vi "multimeterp1.vi"() -> ()   [LabVIEW 2013]
panel:
  in  "Continious \nMeasure":bool
  in  "Measure":bool
  out "Results, V":string[](array[string])
  in  "Range-":bool
  in  "Range+":bool
  out "error out":errorcluster
  in  "Mode":T1(radio)
  out "Range MAX":dbl format="%#_13g"
  out "Range No":dbl format="%#_13g"
  in  "VISA Address":refnum<visa-resource-name>
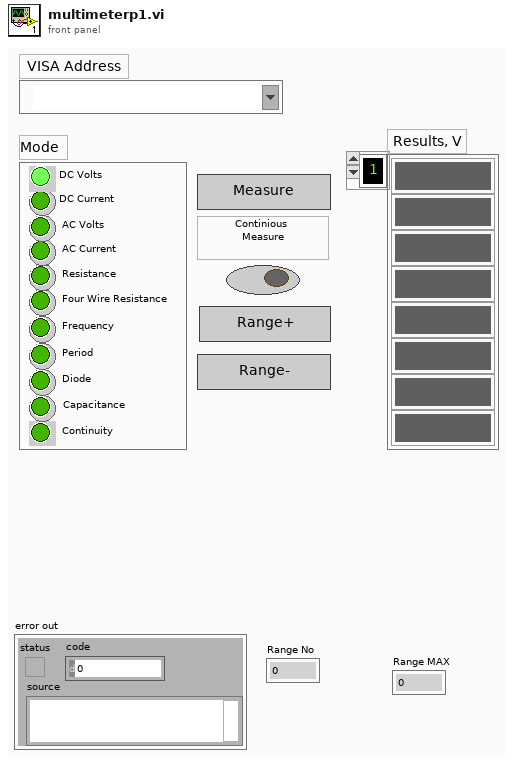
[diagram p1: front panel]
types:
  T1 = enum32{"DC Volts", "DC Current", "AC Volts", "AC Current", "Resistance", "Four Wire Resistance", "Frequency", "Period", "Diode", "Capacitance", "Continuity"}
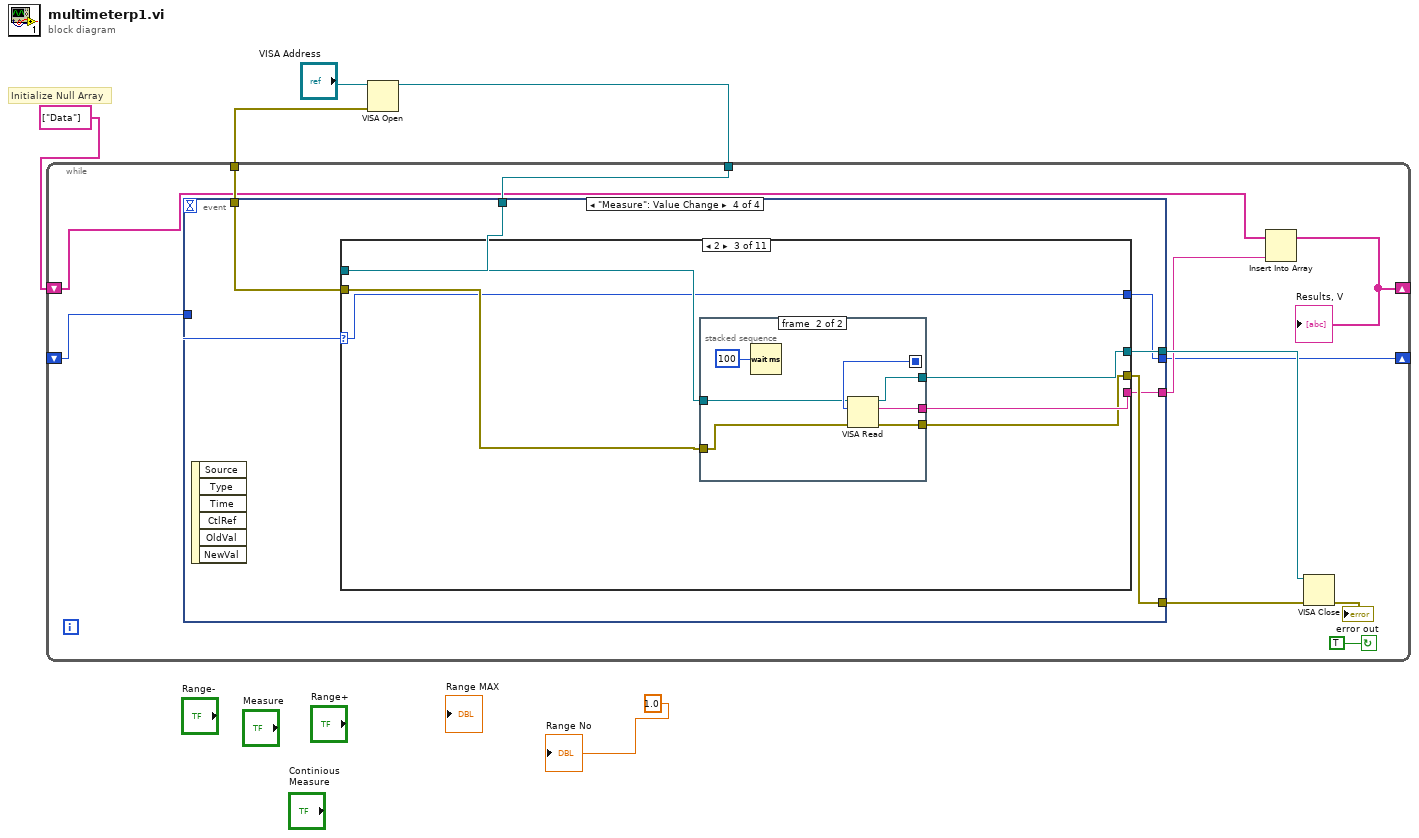
[diagram p0: block diagram]
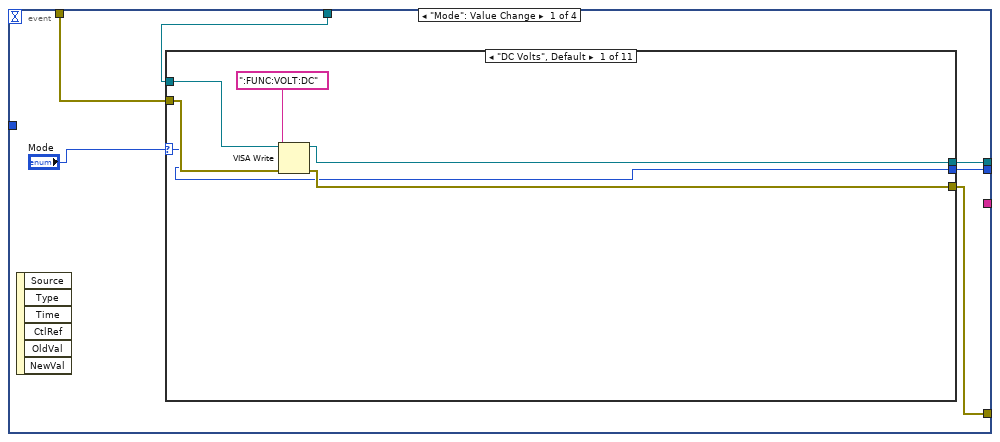
[diagram p2: hidden frame]
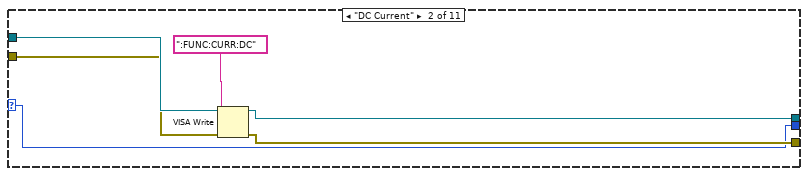
[diagram p3: hidden frame]
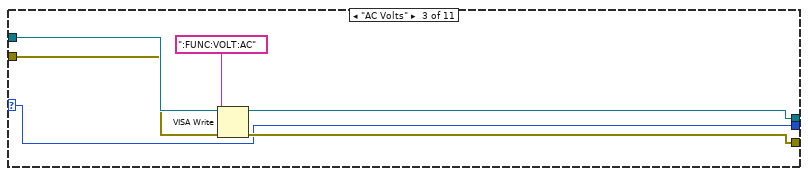
[diagram p4: hidden frame]
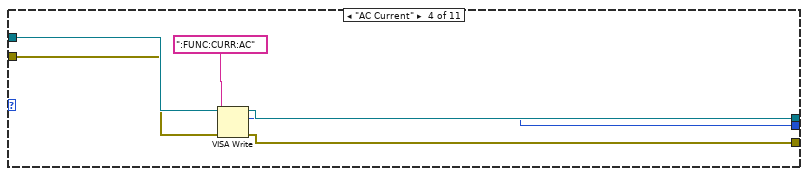
[diagram p5: hidden frame]
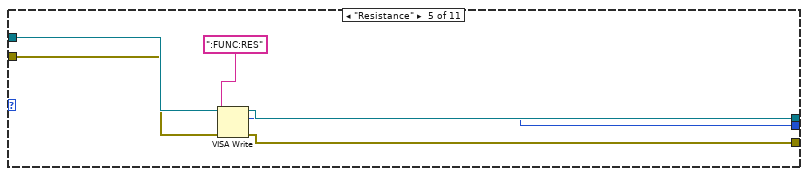
[diagram p6: hidden frame]
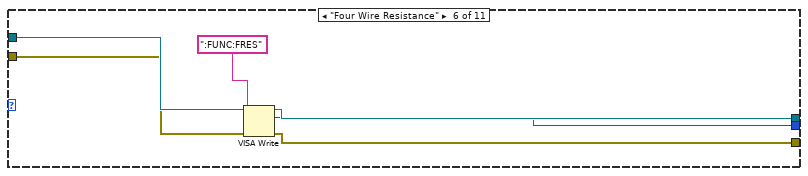
[diagram p7: hidden frame]
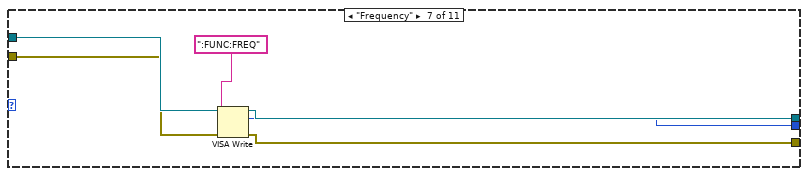
[diagram p8: hidden frame]
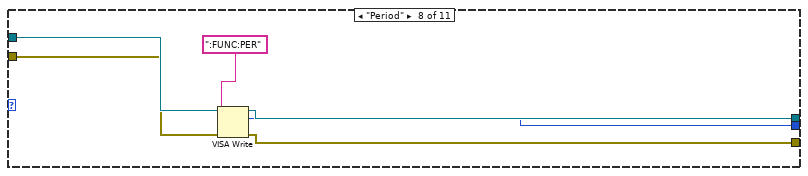
[diagram p9: hidden frame]
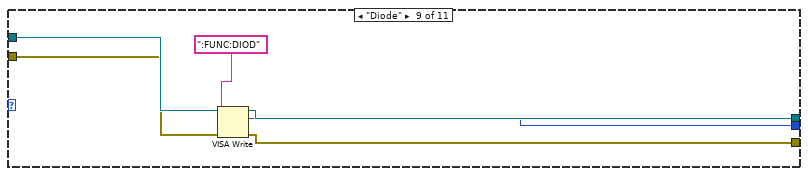
[diagram p10: hidden frame]
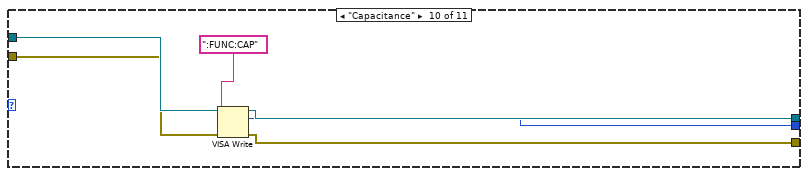
[diagram p11: hidden frame]
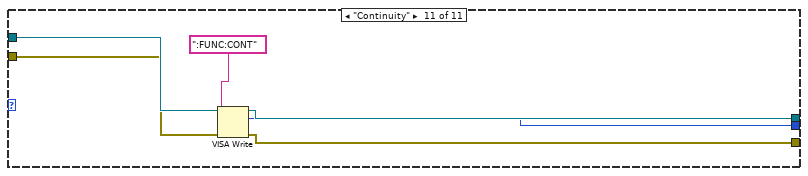
[diagram p12: hidden frame]
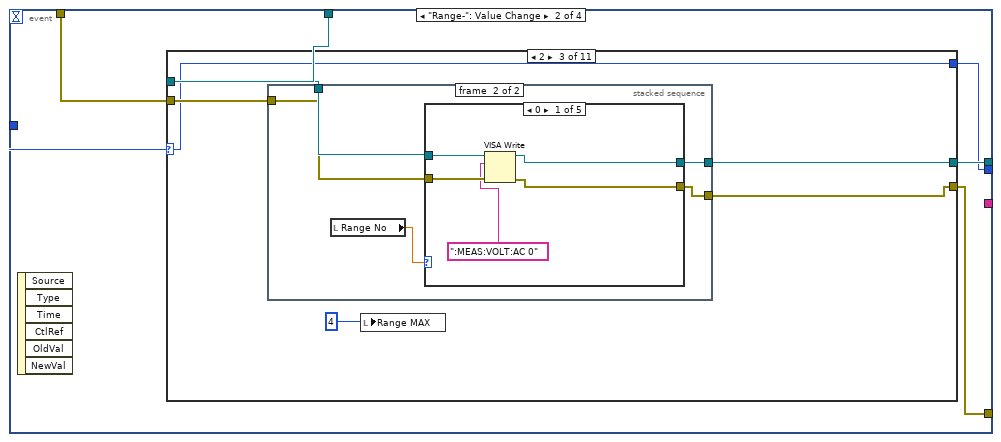
[diagram p13: hidden frame]
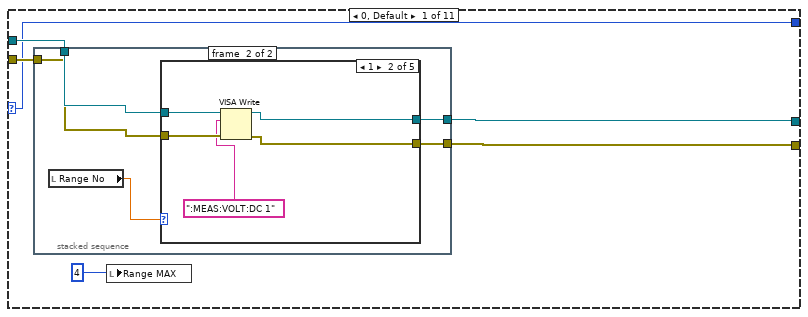
[diagram p14: hidden frame]
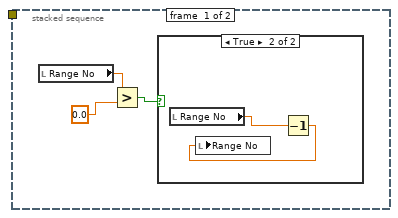
[diagram p15: hidden frame]
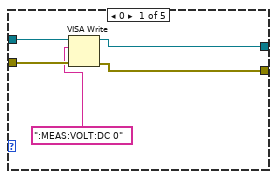
[diagram p17: hidden frame]
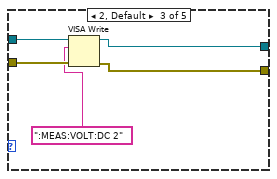
[diagram p18: hidden frame]
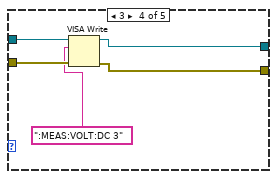
[diagram p19: hidden frame]
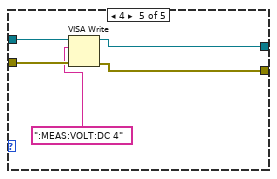
[diagram p20: hidden frame]
diagram:
  # "Initialize Null Array"
  n1 = VISA Open(VISA resource name="VISA Address") -> (VISA resource name=w2:refnum<visa-resource-name>, error out=w3:errorcluster)  [unwired: 4 in]
  n2 = while {
    tunnel: w3 -> [w14]
    tunnel: w2 -> [w13]
    shift-right: [w8] -> _
    shift-left: _ -> [w9]
    shift-right: [w7] -> _
    shift-left: string[] ["Data"] ("array") -> [w6]
    stop <- TRUE continue-if-true
    n3 = event shown="[3] \"Measure\": Value Change" {
      selector: _ -> [_ _ _ _]
      dyn-events: _ -> [_ _ _ _]
      timeout: _ -> [_ _ _ _]
      tunnel: w14 -> [w22 w94 w576 w1059]
      tunnel: w13 -> [w19 w91 w573 w1056]
      tunnel: [w21 w93 w575 w1058] -> w12
      tunnel: [w20 w92 w574 w1057] -> w11
      tunnel: [_ _ _ w1055] -> w10
      tunnel: w9 -> [_ w90 w572 w1054]
      tunnel: [w18 w89 w571 w1053] -> w8
      event "Mode": Value Change {
        n4 = event-data() -> ()  [unwired: 1 in, 6 out]
        n5 = case shown="\"DC Volts\", Default" "Mode" {
          selector: "Mode" -> [w23 w29 w35 _ _ _ _ _ _ _ _]
          tunnel: w19 -> [w26 w33 w39 w45 w51 w57 w63 w69 w75 w81 w87]
          tunnel: w22 -> [w27 w32 w38 w44 w50 w56 w62 w68 w74 w80 w86]
          tunnel: [w24 w30 w36 w42 w48 w54 w60 w66 w72 w78 w84] -> w21
          tunnel: [w25 w31 w37 w43 w49 w55 w61 w67 w73 w79 w85] -> w20
          tunnel: [w23 w29 w35 w41 w47 w53 w59 w65 w71 w77 w83] -> w18
          frame "DC Volts", Default {
            n6 = VISA Write(VISA resource name=w26, write buffer=":FUNC:VOLT:DC", error in (no error)=w27) -> (VISA resource name out=w25:refnum<visa-resource-name>, error out=w24:errorcluster)  [unwired: 1 out]
          }
          frame "DC Current" {
            n7 = VISA Write(VISA resource name=w33, write buffer=":FUNC:CURR:DC", error in (no error)=w32) -> (VISA resource name out=w31:refnum<visa-resource-name>, error out=w30:errorcluster)  [unwired: 1 out]
          }
          frame "AC Volts" {
            n8 = VISA Write(VISA resource name=w39, write buffer=":FUNC:VOLT:AC", error in (no error)=w38) -> (VISA resource name out=w37:refnum<visa-resource-name>, error out=w36:errorcluster)  [unwired: 1 out]
          }
          frame "AC Current" {
            n9 = VISA Write(VISA resource name=w45, write buffer=":FUNC:CURR:AC", error in (no error)=w44) -> (VISA resource name out=w43:refnum<visa-resource-name>, return count=w41:u32, error out=w42:errorcluster)
          }
          frame "Resistance" {
            n10 = VISA Write(VISA resource name=w51, write buffer=":FUNC:RES", error in (no error)=w50) -> (VISA resource name out=w49:refnum<visa-resource-name>, return count=w47:u32, error out=w48:errorcluster)
          }
          frame "Four Wire Resistance" {
            n11 = VISA Write(VISA resource name=w57, write buffer=":FUNC:FRES", error in (no error)=w56) -> (VISA resource name out=w55:refnum<visa-resource-name>, return count=w53:u32, error out=w54:errorcluster)
          }
          frame "Frequency" {
            n12 = VISA Write(VISA resource name=w63, write buffer=":FUNC:FREQ", error in (no error)=w62) -> (VISA resource name out=w61:refnum<visa-resource-name>, return count=w59:u32, error out=w60:errorcluster)
          }
          frame "Period" {
            n13 = VISA Write(VISA resource name=w69, write buffer=":FUNC:PER", error in (no error)=w68) -> (VISA resource name out=w67:refnum<visa-resource-name>, return count=w65:u32, error out=w66:errorcluster)
          }
          frame "Diode" {
            n14 = VISA Write(VISA resource name=w75, write buffer=":FUNC:DIOD", error in (no error)=w74) -> (VISA resource name out=w73:refnum<visa-resource-name>, return count=w71:u32, error out=w72:errorcluster)
          }
          frame "Capacitance" {
            n15 = VISA Write(VISA resource name=w81, write buffer=":FUNC:CAP", error in (no error)=w80) -> (VISA resource name out=w79:refnum<visa-resource-name>, return count=w77:u32, error out=w78:errorcluster)
          }
          frame "Continuity" {
            n16 = VISA Write(VISA resource name=w87, write buffer=":FUNC:CONT", error in (no error)=w86) -> (VISA resource name out=w85:refnum<visa-resource-name>, return count=w83:u32, error out=w84:errorcluster)
          }
        }
      }
      event "Range-": Value Change {
        n17 = event-data() -> ()  [unwired: 1 in, 6 out]
        n18 = case shown="2" w90 {
          selector: w90 -> [w95 w136 w182 w223 w259 w310 w361 w402 w443 w484 w530]
          tunnel: w91 -> [w99 w138 w186 w227 w263 w314 w364 w405 w446 w485 w532]
          tunnel: w94 -> [w98 w137 w185 w226 w262 w313 w365 w406 w447 w486 w531]
          tunnel: [w96 w139 w183 w224 w261 w311 w362 w403 w444 w487 w533] -> w93
          tunnel: [w97 w140 w184 w225 w260 w312 w363 w404 w445 w488 w534] -> w92
          tunnel: [w95 w136 w182 w223 w259 w310 w361 w402 w443 w484 w530] -> w89
          frame 0, Default {
            n19 = stacked-sequence {
              tunnel: w99 -> [_ w109]
              tunnel: w98 -> [_ w108]
              tunnel: [_ w107] -> w97
              tunnel: [_ w106] -> w96
              frame #0 {
                n20 = local read "Range No"() -> (w102:dbl)
                n21 = Greater?(x=w102, y=0.0) -> (0:w101:bool)
                n22 = case shown="True" w101 {
                  frame False {
                  }
                  frame True {
                    n23 = local read "Range No"() -> (w104:dbl)
                    n24 = Decrement(x=w104) -> (x-1=w105:dbl)
                    n25 = local write "Range No"(w105) -> ()
                  }
                }
              }
              frame #1 {
                n26 = local read "Range No"() -> (w110:dbl)
                n27 = case shown="1" w110 {
                  tunnel: w109 -> [w115 w120 w125 w130 w135]
                  tunnel: w108 -> [w114 w119 w124 w129 w134]
                  tunnel: [w112 w117 w122 w127 w132] -> w107
                  tunnel: [w111 w116 w121 w126 w131] -> w106
                  frame 0 {
                    n28 = VISA Write(VISA resource name=w115, write buffer=":MEAS:VOLT:DC 0", error in (no error)=w114) -> (VISA resource name out=w112:refnum<visa-resource-name>, error out=w111:errorcluster)  [unwired: 1 out]
                  }
                  frame 1 {
                    n29 = VISA Write(VISA resource name=w120, write buffer=":MEAS:VOLT:DC 1", error in (no error)=w119) -> (VISA resource name out=w117:refnum<visa-resource-name>, error out=w116:errorcluster)  [unwired: 1 out]
                  }
                  frame 2, Default {
                    n30 = VISA Write(VISA resource name=w125, write buffer=":MEAS:VOLT:DC 2", error in (no error)=w124) -> (VISA resource name out=w122:refnum<visa-resource-name>, error out=w121:errorcluster)  [unwired: 1 out]
                  }
                  frame 3 {
                    n31 = VISA Write(VISA resource name=w130, write buffer=":MEAS:VOLT:DC 3", error in (no error)=w129) -> (VISA resource name out=w127:refnum<visa-resource-name>, error out=w126:errorcluster)  [unwired: 1 out]
                  }
                  frame 4 {
                    n32 = VISA Write(VISA resource name=w135, write buffer=":MEAS:VOLT:DC 4", error in (no error)=w134) -> (VISA resource name out=w132:refnum<visa-resource-name>, error out=w131:errorcluster)  [unwired: 1 out]
                  }
                }
              }
            }
            n33 = local write "Range MAX"(4) -> ()
          }
          frame 1 {
            n34 = stacked-sequence {
              tunnel: [_ w150] -> w140
              tunnel: [_ w149] -> w139
              tunnel: w138 -> [_ w148]
              tunnel: w137 -> [_ w147]
              frame #0 {
                n35 = local read "Range No"() -> (w143:dbl)
                n36 = Greater?(x=w143, y=0.0) -> (0:w142:bool)
                n37 = case shown="True" w142 {
                  frame False {
                  }
                  frame True {
                    n38 = local read "Range No"() -> (w145:dbl)
                    n39 = Decrement(x=w145) -> (x-1=w146:dbl)
                    n40 = local write "Range No"(w146) -> ()
                  }
                }
              }
              frame #1 {
                n41 = local read "Range No"() -> (w151:dbl)
                n42 = case shown="1" w151 {
                  tunnel: w148 -> [w156 w161 w166 w171 w176 w181]
                  tunnel: w147 -> [w155 w160 w165 w170 w175 w180]
                  tunnel: [w153 w158 w163 w168 w173 w178] -> w150
                  tunnel: [w152 w157 w162 w167 w172 w177] -> w149
                  frame 0 {
                    n43 = VISA Write(VISA resource name=w156, write buffer=":MEAS:CURR:DC 0", error in (no error)=w155) -> (VISA resource name out=w153:refnum<visa-resource-name>, error out=w152:errorcluster)  [unwired: 1 out]
                  }
                  frame 1 {
                    n44 = VISA Write(VISA resource name=w161, write buffer=":MEAS:CURR:DC 1", error in (no error)=w160) -> (VISA resource name out=w158:refnum<visa-resource-name>, error out=w157:errorcluster)  [unwired: 1 out]
                  }
                  frame 2, Default {
                    n45 = VISA Write(VISA resource name=w166, write buffer=":MEAS:CURR:DC 2", error in (no error)=w165) -> (VISA resource name out=w163:refnum<visa-resource-name>, error out=w162:errorcluster)  [unwired: 1 out]
                  }
                  frame 3 {
                    n46 = VISA Write(VISA resource name=w171, write buffer=":MEAS:CURR:DC 3", error in (no error)=w170) -> (VISA resource name out=w168:refnum<visa-resource-name>, error out=w167:errorcluster)  [unwired: 1 out]
                  }
                  frame 4 {
                    n47 = VISA Write(VISA resource name=w176, write buffer=":MEAS:CURR:DC 4", error in (no error)=w175) -> (VISA resource name out=w173:refnum<visa-resource-name>, error out=w172:errorcluster)  [unwired: 1 out]
                  }
                  frame 5 {
                    n48 = VISA Write(VISA resource name=w181, write buffer=":MEAS:CURR:DC 5", error in (no error)=w180) -> (VISA resource name out=w178:refnum<visa-resource-name>, error out=w177:errorcluster)  [unwired: 1 out]
                  }
                }
              }
            }
            n49 = local write "Range MAX"(5) -> ()
          }
          frame 2 {
            n50 = stacked-sequence {
              tunnel: w186 -> [_ w196]
              tunnel: w185 -> [_ w195]
              tunnel: [_ w194] -> w184
              tunnel: [_ w193] -> w183
              frame #0 {
                n51 = local read "Range No"() -> (w189:dbl)
                n52 = Greater?(x=w189, y=0.0) -> (0:w188:bool)
                n53 = case shown="True" w188 {
                  frame False {
                  }
                  frame True {
                    n54 = local read "Range No"() -> (w191:dbl)
                    n55 = Decrement(x=w191) -> (x-1=w192:dbl)
                    n56 = local write "Range No"(w192) -> ()
                  }
                }
              }
              frame #1 {
                n57 = local read "Range No"() -> (w197:dbl)
                n58 = case shown="0" w197 {
                  tunnel: w196 -> [w202 w207 w212 w217 w222]
                  tunnel: w195 -> [w201 w206 w211 w216 w221]
                  tunnel: [w199 w204 w209 w214 w219] -> w194
                  tunnel: [w198 w203 w208 w213 w218] -> w193
                  frame 0 {
                    n59 = VISA Write(VISA resource name=w202, write buffer=":MEAS:VOLT:AC 0", error in (no error)=w201) -> (VISA resource name out=w199:refnum<visa-resource-name>, error out=w198:errorcluster)  [unwired: 1 out]
                  }
                  frame 1 {
                    n60 = VISA Write(VISA resource name=w207, write buffer=":MEAS:VOLT:AC 1", error in (no error)=w206) -> (VISA resource name out=w204:refnum<visa-resource-name>, error out=w203:errorcluster)  [unwired: 1 out]
                  }
                  frame 2, Default {
                    n61 = VISA Write(VISA resource name=w212, write buffer=":MEAS:VOLT:AC 2", error in (no error)=w211) -> (VISA resource name out=w209:refnum<visa-resource-name>, error out=w208:errorcluster)  [unwired: 1 out]
                  }
                  frame 3 {
                    n62 = VISA Write(VISA resource name=w217, write buffer=":MEAS:VOLT:AC 3", error in (no error)=w216) -> (VISA resource name out=w214:refnum<visa-resource-name>, error out=w213:errorcluster)  [unwired: 1 out]
                  }
                  frame 4 {
                    n63 = VISA Write(VISA resource name=w222, write buffer=":MEAS:VOLT:AC 4", error in (no error)=w221) -> (VISA resource name out=w219:refnum<visa-resource-name>, error out=w218:errorcluster)  [unwired: 1 out]
                  }
                }
              }
            }
            n64 = local write "Range MAX"(4) -> ()
          }
          frame 3 {
            n65 = stacked-sequence {
              tunnel: w227 -> [_ w237]
              tunnel: w226 -> [_ w236]
              tunnel: [_ w235] -> w225
              tunnel: [_ w234] -> w224
              frame #0 {
                n66 = local read "Range No"() -> (w230:dbl)
                n67 = Greater?(x=w230, y=0.0) -> (0:w229:bool)
                n68 = case shown="True" w229 {
                  frame False {
                  }
                  frame True {
                    n69 = local read "Range No"() -> (w232:dbl)
                    n70 = Decrement(x=w232) -> (x-1=w233:dbl)
                    n71 = local write "Range No"(w233) -> ()
                  }
                }
              }
              frame #1 {
                n72 = local read "Range No"() -> (w238:dbl)
                n73 = case shown="0" w238 {
                  tunnel: w237 -> [w243 w248 w253 w258]
                  tunnel: w236 -> [w242 w247 w252 w257]
                  tunnel: [w240 w245 w250 w255] -> w235
                  tunnel: [w239 w244 w249 w254] -> w234
                  frame 0 {
                    n74 = VISA Write(VISA resource name=w243, write buffer=":MEAS:CURR:AC 0", error in (no error)=w242) -> (VISA resource name out=w240:refnum<visa-resource-name>, error out=w239:errorcluster)  [unwired: 1 out]
                  }
                  frame 1 {
                    n75 = VISA Write(VISA resource name=w248, write buffer=":MEAS:CURR:AC 1", error in (no error)=w247) -> (VISA resource name out=w245:refnum<visa-resource-name>, error out=w244:errorcluster)  [unwired: 1 out]
                  }
                  frame 2, Default {
                    n76 = VISA Write(VISA resource name=w253, write buffer=":MEAS:CURR:AC 2", error in (no error)=w252) -> (VISA resource name out=w250:refnum<visa-resource-name>, error out=w249:errorcluster)  [unwired: 1 out]
                  }
                  frame 3 {
                    n77 = VISA Write(VISA resource name=w258, write buffer=":MEAS:CURR:AC 3", error in (no error)=w257) -> (VISA resource name out=w255:refnum<visa-resource-name>, error out=w254:errorcluster)  [unwired: 1 out]
                  }
                }
              }
            }
            n78 = local write "Range MAX"(3) -> ()
          }
          frame 4 {
            n79 = stacked-sequence {
              tunnel: w263 -> [_ w273]
              tunnel: w262 -> [_ w272]
              tunnel: [_ w271] -> w261
              tunnel: [_ w270] -> w260
              frame #0 {
                n80 = local read "Range No"() -> (w266:dbl)
                n81 = Greater?(x=w266, y=0.0) -> (0:w265:bool)
                n82 = case shown="True" w265 {
                  frame False {
                  }
                  frame True {
                    n83 = local read "Range No"() -> (w268:dbl)
                    n84 = Decrement(x=w268) -> (x-1=w269:dbl)
                    n85 = local write "Range No"(w269) -> ()
                  }
                }
              }
              frame #1 {
                n86 = local read "Range No"() -> (w274:dbl)
                n87 = case shown="1" w274 {
                  tunnel: w273 -> [w279 w284 w289 w294 w299 w304 w309]
                  tunnel: w272 -> [w278 w283 w288 w293 w298 w303 w308]
                  tunnel: [w276 w281 w286 w291 w296 w301 w306] -> w270
                  tunnel: [w275 w280 w285 w290 w295 w300 w305] -> w271
                  frame 0 {
                    n88 = VISA Write(VISA resource name=w279, write buffer=":MEAS:RES 0", error in (no error)=w278) -> (VISA resource name out=w276:refnum<visa-resource-name>, error out=w275:errorcluster)  [unwired: 1 out]
                  }
                  frame 1 {
                    n89 = VISA Write(VISA resource name=w284, write buffer=":MEAS:RES 1", error in (no error)=w283) -> (VISA resource name out=w281:refnum<visa-resource-name>, error out=w280:errorcluster)  [unwired: 1 out]
                  }
                  frame 2, Default {
                    n90 = VISA Write(VISA resource name=w289, write buffer=":MEAS:RES 2", error in (no error)=w288) -> (VISA resource name out=w286:refnum<visa-resource-name>, error out=w285:errorcluster)  [unwired: 1 out]
                  }
                  frame 3 {
                    n91 = VISA Write(VISA resource name=w294, write buffer=":MEAS:RES 3", error in (no error)=w293) -> (VISA resource name out=w291:refnum<visa-resource-name>, error out=w290:errorcluster)  [unwired: 1 out]
                  }
                  frame 4 {
                    n92 = VISA Write(VISA resource name=w299, write buffer=":MEAS:RES 4", error in (no error)=w298) -> (VISA resource name out=w296:refnum<visa-resource-name>, error out=w295:errorcluster)  [unwired: 1 out]
                  }
                  frame 5 {
                    n93 = VISA Write(VISA resource name=w304, write buffer=":MEAS:RES 5", error in (no error)=w303) -> (VISA resource name out=w301:refnum<visa-resource-name>, error out=w300:errorcluster)  [unwired: 1 out]
                  }
                  frame 6 {
                    n94 = VISA Write(VISA resource name=w309, write buffer=":MEAS:RES 6", error in (no error)=w308) -> (VISA resource name out=w306:refnum<visa-resource-name>, error out=w305:errorcluster)  [unwired: 1 out]
                  }
                }
              }
            }
            n95 = local write "Range MAX"(6) -> ()
          }
          frame 5 {
            n96 = stacked-sequence {
              tunnel: w314 -> [_ w324]
              tunnel: w313 -> [_ w323]
              tunnel: [_ w322] -> w312
              tunnel: [_ w321] -> w311
              frame #0 {
                n97 = local read "Range No"() -> (w317:dbl)
                n98 = Greater?(x=w317, y=0.0) -> (0:w316:bool)
                n99 = case shown="True" w316 {
                  frame False {
                  }
                  frame True {
                    n100 = local read "Range No"() -> (w319:dbl)
                    n101 = Decrement(x=w319) -> (x-1=w320:dbl)
                    n102 = local write "Range No"(w320) -> ()
                  }
                }
              }
              frame #1 {
                n103 = local read "Range No"() -> (w325:dbl)
                n104 = case shown="6" w325 {
                  tunnel: w324 -> [w330 w335 w340 w345 w350 w355 w360]
                  tunnel: w323 -> [w329 w334 w339 w344 w349 w354 w359]
                  tunnel: [w327 w332 w337 w342 w347 w352 w357] -> w322
                  tunnel: [w326 w331 w336 w341 w346 w351 w356] -> w321
                  frame 0 {
                    n105 = VISA Write(VISA resource name=w330, write buffer=":MEAS:FRES 0", error in (no error)=w329) -> (VISA resource name out=w327:refnum<visa-resource-name>, error out=w326:errorcluster)  [unwired: 1 out]
                  }
                  frame 1 {
                    n106 = VISA Write(VISA resource name=w335, write buffer=":MEAS:FRES 1", error in (no error)=w334) -> (VISA resource name out=w332:refnum<visa-resource-name>, error out=w331:errorcluster)  [unwired: 1 out]
                  }
                  frame 2, Default {
                    n107 = VISA Write(VISA resource name=w340, write buffer=":MEAS:FRES 2", error in (no error)=w339) -> (VISA resource name out=w337:refnum<visa-resource-name>, error out=w336:errorcluster)  [unwired: 1 out]
                  }
                  frame 3 {
                    n108 = VISA Write(VISA resource name=w345, write buffer=":MEAS:FRES 3", error in (no error)=w344) -> (VISA resource name out=w342:refnum<visa-resource-name>, error out=w341:errorcluster)  [unwired: 1 out]
                  }
                  frame 4 {
                    n109 = VISA Write(VISA resource name=w350, write buffer=":MEAS:FRES 4", error in (no error)=w349) -> (VISA resource name out=w347:refnum<visa-resource-name>, error out=w346:errorcluster)  [unwired: 1 out]
                  }
                  frame 5 {
                    n110 = VISA Write(VISA resource name=w355, write buffer=":MEAS:FRES 5", error in (no error)=w354) -> (VISA resource name out=w352:refnum<visa-resource-name>, error out=w351:errorcluster)  [unwired: 1 out]
                  }
                  frame 6 {
                    n111 = VISA Write(VISA resource name=w360, write buffer=":MEAS:FRES 6", error in (no error)=w359) -> (VISA resource name out=w357:refnum<visa-resource-name>, error out=w356:errorcluster)  [unwired: 1 out]
                  }
                }
              }
            }
            n112 = local write "Range MAX"(6) -> ()
          }
          frame 6 {
            n113 = stacked-sequence {
              tunnel: w365 -> [_ w375]
              tunnel: w364 -> [_ w374]
              tunnel: [_ w373] -> w363
              tunnel: [_ w372] -> w362
              frame #0 {
                n114 = local read "Range No"() -> (w368:dbl)
                n115 = Greater?(x=w368, y=0.0) -> (0:w367:bool)
                n116 = case shown="True" w367 {
                  frame False {
                  }
                  frame True {
                    n117 = local read "Range No"() -> (w370:dbl)
                    n118 = Decrement(x=w370) -> (x-1=w371:dbl)
                    n119 = local write "Range No"(w371) -> ()
                  }
                }
              }
              frame #1 {
                n120 = local read "Range No"() -> (w376:dbl)
                n121 = case shown="1" w376 {
                  tunnel: w374 -> [w381 w386 w391 w396 w401]
                  tunnel: w375 -> [w380 w385 w390 w395 w400]
                  tunnel: [w378 w383 w388 w393 w398] -> w373
                  tunnel: [w377 w382 w387 w392 w397] -> w372
                  frame 0 {
                    n122 = VISA Write(VISA resource name=w381, write buffer=":MEAS:FREQ 0", error in (no error)=w380) -> (VISA resource name out=w378:refnum<visa-resource-name>, error out=w377:errorcluster)  [unwired: 1 out]
                  }
                  frame 1 {
                    n123 = VISA Write(VISA resource name=w386, write buffer=":MEAS:FREQ 1", error in (no error)=w385) -> (VISA resource name out=w383:refnum<visa-resource-name>, error out=w382:errorcluster)  [unwired: 1 out]
                  }
                  frame 2, Default {
                    n124 = VISA Write(VISA resource name=w391, write buffer=":MEAS:FREQ 2", error in (no error)=w390) -> (VISA resource name out=w388:refnum<visa-resource-name>, error out=w387:errorcluster)  [unwired: 1 out]
                  }
                  frame 3 {
                    n125 = VISA Write(VISA resource name=w396, write buffer=":MEAS:FREQ 3", error in (no error)=w395) -> (VISA resource name out=w393:refnum<visa-resource-name>, error out=w392:errorcluster)  [unwired: 1 out]
                  }
                  frame 4 {
                    n126 = VISA Write(VISA resource name=w401, write buffer=":MEAS:FREQ 4", error in (no error)=w400) -> (VISA resource name out=w398:refnum<visa-resource-name>, error out=w397:errorcluster)  [unwired: 1 out]
                  }
                }
              }
            }
            n127 = local write "Range MAX"(4) -> ()
          }
          frame 7 {
            n128 = stacked-sequence {
              tunnel: w406 -> [_ w416]
              tunnel: w405 -> [_ w415]
              tunnel: [_ w414] -> w404
              tunnel: [_ w413] -> w403
              frame #0 {
                n129 = local read "Range No"() -> (w409:dbl)
                n130 = Greater?(x=w409, y=0.0) -> (0:w408:bool)
                n131 = case shown="True" w408 {
                  frame False {
                  }
                  frame True {
                    n132 = local read "Range No"() -> (w411:dbl)
                    n133 = Decrement(x=w411) -> (x-1=w412:dbl)
                    n134 = local write "Range No"(w412) -> ()
                  }
                }
              }
              frame #1 {
                n135 = local read "Range No"() -> (w417:dbl)
                n136 = case shown="0" w417 {
                  tunnel: w415 -> [w422 w427 w432 w437 w442]
                  tunnel: w416 -> [w421 w426 w431 w436 w441]
                  tunnel: [w419 w424 w429 w434 w439] -> w414
                  tunnel: [w418 w423 w428 w433 w438] -> w413
                  frame 0 {
                    n137 = VISA Write(VISA resource name=w422, write buffer=":MEAS:PER 0", error in (no error)=w421) -> (VISA resource name out=w419:refnum<visa-resource-name>, error out=w418:errorcluster)  [unwired: 1 out]
                  }
                  frame 1 {
                    n138 = VISA Write(VISA resource name=w427, write buffer=":MEAS:PER 1", error in (no error)=w426) -> (VISA resource name out=w424:refnum<visa-resource-name>, error out=w423:errorcluster)  [unwired: 1 out]
                  }
                  frame 2, Default {
                    n139 = VISA Write(VISA resource name=w432, write buffer=":MEAS:PER 2", error in (no error)=w431) -> (VISA resource name out=w429:refnum<visa-resource-name>, error out=w428:errorcluster)  [unwired: 1 out]
                  }
                  frame 3 {
                    n140 = VISA Write(VISA resource name=w437, write buffer=":MEAS:PER 3", error in (no error)=w436) -> (VISA resource name out=w434:refnum<visa-resource-name>, error out=w433:errorcluster)  [unwired: 1 out]
                  }
                  frame 4 {
                    n141 = VISA Write(VISA resource name=w442, write buffer=":MEAS:PER 4", error in (no error)=w441) -> (VISA resource name out=w439:refnum<visa-resource-name>, error out=w438:errorcluster)  [unwired: 1 out]
                  }
                }
              }
            }
            n142 = local write "Range MAX"(4) -> ()
          }
          frame 8 {
            n143 = stacked-sequence {
              tunnel: w447 -> [_ w457]
              tunnel: w446 -> [_ w456]
              tunnel: [_ w455] -> w445
              tunnel: [_ w454] -> w444
              frame #0 {
                n144 = local read "Range No"() -> (w450:dbl)
                n145 = Greater?(x=w450, y=0.0) -> (0:w449:bool)
                n146 = case shown="True" w449 {
                  frame False {
                  }
                  frame True {
                    n147 = local read "Range No"() -> (w452:dbl)
                    n148 = Decrement(x=w452) -> (x-1=w453:dbl)
                    n149 = local write "Range No"(w453) -> ()
                  }
                }
              }
              frame #1 {
                n150 = local read "Range No"() -> (w458:dbl)
                n151 = case shown="0" w458 {
                  tunnel: w456 -> [w463 w468 w473 w478 w483]
                  tunnel: w457 -> [w462 w467 w472 w477 w482]
                  tunnel: [w460 w465 w470 w475 w480] -> w455
                  tunnel: [w459 w464 w469 w474 w479] -> w454
                  frame 0 {
                    n152 = VISA Write(VISA resource name=w463, write buffer=":MEAS:VOLT:DC 0", error in (no error)=w462) -> (VISA resource name out=w460:refnum<visa-resource-name>, error out=w459:errorcluster)  [unwired: 1 out]
                  }
                  frame 1 {
                    n153 = VISA Write(VISA resource name=w468, write buffer=":MEAS:VOLT:DC 1", error in (no error)=w467) -> (VISA resource name out=w465:refnum<visa-resource-name>, error out=w464:errorcluster)  [unwired: 1 out]
                  }
                  frame 2, Default {
                    n154 = VISA Write(VISA resource name=w473, write buffer=":MEAS:VOLT:DC 2", error in (no error)=w472) -> (VISA resource name out=w470:refnum<visa-resource-name>, error out=w469:errorcluster)  [unwired: 1 out]
                  }
                  frame 3 {
                    n155 = VISA Write(VISA resource name=w478, write buffer=":MEAS:VOLT:DC 3", error in (no error)=w477) -> (VISA resource name out=w475:refnum<visa-resource-name>, error out=w474:errorcluster)  [unwired: 1 out]
                  }
                  frame 4 {
                    n156 = VISA Write(VISA resource name=w483, write buffer=":MEAS:VOLT:DC 4", error in (no error)=w482) -> (VISA resource name out=w480:refnum<visa-resource-name>, error out=w479:errorcluster)  [unwired: 1 out]
                  }
                }
              }
            }
            n157 = local write "Range MAX"(4) -> ()
          }
          frame 9 {
            n158 = stacked-sequence {
              tunnel: [_ w498] -> w488
              tunnel: [_ w497] -> w487
              tunnel: w486 -> [_ w496]
              tunnel: w485 -> [_ w495]
              frame #0 {
                n159 = local read "Range No"() -> (w491:dbl)
                n160 = Greater?(x=w491, y=0.0) -> (0:w490:bool)
                n161 = case shown="True" w490 {
                  frame False {
                  }
                  frame True {
                    n162 = local read "Range No"() -> (w493:dbl)
                    n163 = Decrement(x=w493) -> (x-1=w494:dbl)
                    n164 = local write "Range No"(w494) -> ()
                  }
                }
              }
              frame #1 {
                n165 = local read "Range No"() -> (w499:dbl)
                n166 = case shown="5" w499 {
                  tunnel: w495 -> [w504 w509 w514 w519 w524 w529]
                  tunnel: w496 -> [w503 w508 w513 w518 w523 w528]
                  tunnel: [w501 w506 w511 w516 w521 w526] -> w498
                  tunnel: [w500 w505 w510 w515 w520 w525] -> w497
                  frame 0 {
                    n167 = VISA Write(VISA resource name=w504, write buffer=":MEAS:CAP 0", error in (no error)=w503) -> (VISA resource name out=w501:refnum<visa-resource-name>, error out=w500:errorcluster)  [unwired: 1 out]
                  }
                  frame 1 {
                    n168 = VISA Write(VISA resource name=w509, write buffer=":MEAS:CAP 1", error in (no error)=w508) -> (VISA resource name out=w506:refnum<visa-resource-name>, error out=w505:errorcluster)  [unwired: 1 out]
                  }
                  frame 2, Default {
                    n169 = VISA Write(VISA resource name=w514, write buffer=":MEAS:CAP 2", error in (no error)=w513) -> (VISA resource name out=w511:refnum<visa-resource-name>, error out=w510:errorcluster)  [unwired: 1 out]
                  }
                  frame 3 {
                    n170 = VISA Write(VISA resource name=w519, write buffer=":MEAS:CAP 3", error in (no error)=w518) -> (VISA resource name out=w516:refnum<visa-resource-name>, error out=w515:errorcluster)  [unwired: 1 out]
                  }
                  frame 4 {
                    n171 = VISA Write(VISA resource name=w524, write buffer=":MEAS:CAP 4", error in (no error)=w523) -> (VISA resource name out=w521:refnum<visa-resource-name>, error out=w520:errorcluster)  [unwired: 1 out]
                  }
                  frame 5 {
                    n172 = VISA Write(VISA resource name=w529, write buffer=":MEAS:CAP 5", error in (no error)=w528) -> (VISA resource name out=w526:refnum<visa-resource-name>, error out=w525:errorcluster)  [unwired: 1 out]
                  }
                }
              }
            }
            n173 = local write "Range MAX"(5) -> ()
          }
          frame 10 {
            n174 = stacked-sequence {
              tunnel: [_ w544] -> w534
              tunnel: [_ w543] -> w533
              tunnel: w532 -> [_ w542]
              tunnel: w531 -> [_ w541]
              frame #0 {
                n175 = local read "Range No"() -> (w537:dbl)
                n176 = Greater?(x=w537, y=0.0) -> (0:w536:bool)
                n177 = case shown="True" w536 {
                  frame False {
                  }
                  frame True {
                    n178 = local read "Range No"() -> (w539:dbl)
                    n179 = Decrement(x=w539) -> (x-1=w540:dbl)
                    n180 = local write "Range No"(w540) -> ()
                  }
                }
              }
              frame #1 {
                n181 = local read "Range No"() -> (w545:dbl)
                n182 = case shown="2, Default" w545 {
                  tunnel: w542 -> [w550 w555 w560 w565 w570]
                  tunnel: w541 -> [w549 w554 w559 w564 w569]
                  tunnel: [w547 w552 w557 w562 w567] -> w544
                  tunnel: [w546 w551 w556 w561 w566] -> w543
                  frame 0 {
                    n183 = VISA Write(VISA resource name=w550, write buffer=":MEAS:VOLT:DC 0", error in (no error)=w549) -> (VISA resource name out=w547:refnum<visa-resource-name>, error out=w546:errorcluster)  [unwired: 1 out]
                  }
                  frame 1 {
                    n184 = VISA Write(VISA resource name=w555, write buffer=":MEAS:VOLT:DC 1", error in (no error)=w554) -> (VISA resource name out=w552:refnum<visa-resource-name>, error out=w551:errorcluster)  [unwired: 1 out]
                  }
                  frame 2, Default {
                    n185 = VISA Write(VISA resource name=w560, write buffer=":MEAS:VOLT:DC 2", error in (no error)=w559) -> (VISA resource name out=w557:refnum<visa-resource-name>, error out=w556:errorcluster)  [unwired: 1 out]
                  }
                  frame 3 {
                    n186 = VISA Write(VISA resource name=w565, write buffer=":MEAS:VOLT:DC 3", error in (no error)=w564) -> (VISA resource name out=w562:refnum<visa-resource-name>, error out=w561:errorcluster)  [unwired: 1 out]
                  }
                  frame 4 {
                    n187 = VISA Write(VISA resource name=w570, write buffer=":MEAS:VOLT:DC 4", error in (no error)=w569) -> (VISA resource name out=w567:refnum<visa-resource-name>, error out=w566:errorcluster)  [unwired: 1 out]
                  }
                }
              }
            }
            n188 = local write "Range MAX"(4) -> ()
          }
        }
      }
      event "Range+": Value Change {
        n189 = event-data() -> ()  [unwired: 1 in, 6 out]
        n190 = case shown="9" w572 {
          selector: w572 -> [w577 w618 w664 w705 w741 w792 w843 w884 w925 w966 w1012]
          tunnel: w573 -> [w581 w620 w668 w709 w745 w796 w846 w887 w928 w967 w1014]
          tunnel: w576 -> [w580 w619 w667 w708 w744 w795 w847 w888 w929 w968 w1013]
          tunnel: [w578 w621 w665 w706 w743 w793 w844 w885 w926 w969 w1015] -> w575
          tunnel: [w579 w622 w666 w707 w742 w794 w845 w886 w927 w970 w1016] -> w574
          tunnel: [w577 w618 w664 w705 w741 w792 w843 w884 w925 w966 w1012] -> w571
          frame 0, Default {
            n191 = stacked-sequence {
              tunnel: w581 -> [_ w591]
              tunnel: w580 -> [_ w590]
              tunnel: [_ w589] -> w579
              tunnel: [_ w588] -> w578
              frame #0 {
                n192 = local read "Range MAX"() -> (w583:dbl)
                n193 = local read "Range No"() -> (w584:dbl)
                n194 = Less?(x=w584, y=w583) -> (x < y?=w585:bool)
                n195 = case shown="True" w585 {
                  frame False {
                  }
                  frame True {
                    n196 = local read "Range No"() -> (w587:dbl)
                    n197 = Increment(x=w587) -> (x+1=w586:dbl)
                    n198 = local write "Range No"(w586) -> ()
                  }
                }
              }
              frame #1 {
                n199 = local read "Range No"() -> (w592:dbl)
                n200 = case shown="2, Default" w592 {
                  tunnel: w591 -> [w597 w602 w607 w612 w617]
                  tunnel: w590 -> [w596 w601 w606 w611 w616]
                  tunnel: [w594 w599 w604 w609 w614] -> w589
                  tunnel: [w593 w598 w603 w608 w613] -> w588
                  frame 0 {
                    n201 = VISA Write(VISA resource name=w597, write buffer=":MEAS:VOLT:DC 0", error in (no error)=w596) -> (VISA resource name out=w594:refnum<visa-resource-name>, error out=w593:errorcluster)  [unwired: 1 out]
                  }
                  frame 1 {
                    n202 = VISA Write(VISA resource name=w602, write buffer=":MEAS:VOLT:DC 1", error in (no error)=w601) -> (VISA resource name out=w599:refnum<visa-resource-name>, error out=w598:errorcluster)  [unwired: 1 out]
                  }
                  frame 2, Default {
                    n203 = VISA Write(VISA resource name=w607, write buffer=":MEAS:VOLT:DC 2", error in (no error)=w606) -> (VISA resource name out=w604:refnum<visa-resource-name>, error out=w603:errorcluster)  [unwired: 1 out]
                  }
                  frame 3 {
                    n204 = VISA Write(VISA resource name=w612, write buffer=":MEAS:VOLT:DC 3", error in (no error)=w611) -> (VISA resource name out=w609:refnum<visa-resource-name>, error out=w608:errorcluster)  [unwired: 1 out]
                  }
                  frame 4 {
                    n205 = VISA Write(VISA resource name=w617, write buffer=":MEAS:VOLT:DC 4", error in (no error)=w616) -> (VISA resource name out=w614:refnum<visa-resource-name>, error out=w613:errorcluster)  [unwired: 1 out]
                  }
                }
              }
            }
            n206 = local write "Range MAX"(4) -> ()
          }
          frame 1 {
            n207 = stacked-sequence {
              tunnel: [_ w632] -> w622
              tunnel: [_ w631] -> w621
              tunnel: w620 -> [_ w630]
              tunnel: w619 -> [_ w629]
              frame #0 {
                n208 = local read "Range MAX"() -> (w626:dbl)
                n209 = local read "Range No"() -> (w625:dbl)
                n210 = Less?(x=w625, y=w626) -> (x < y?=w624:bool)
                n211 = case shown="True" w624 {
                  frame False {
                  }
                  frame True {
                    n212 = local read "Range No"() -> (w628:dbl)
                    n213 = Increment(x=w628) -> (x+1=w627:dbl)
                    n214 = local write "Range No"(w627) -> ()
                  }
                }
              }
              frame #1 {
                n215 = local read "Range No"() -> (w633:dbl)
                n216 = case shown="2, Default" w633 {
                  tunnel: w630 -> [w638 w643 w648 w653 w658 w663]
                  tunnel: w629 -> [w637 w642 w647 w652 w657 w662]
                  tunnel: [w635 w640 w645 w650 w655 w660] -> w632
                  tunnel: [w634 w639 w644 w649 w654 w659] -> w631
                  frame 0 {
                    n217 = VISA Write(VISA resource name=w638, write buffer=":MEAS:CURR:DC 0", error in (no error)=w637) -> (VISA resource name out=w635:refnum<visa-resource-name>, error out=w634:errorcluster)  [unwired: 1 out]
                  }
                  frame 1 {
                    n218 = VISA Write(VISA resource name=w643, write buffer=":MEAS:CURR:DC 1", error in (no error)=w642) -> (VISA resource name out=w640:refnum<visa-resource-name>, error out=w639:errorcluster)  [unwired: 1 out]
                  }
                  frame 2, Default {
                    n219 = VISA Write(VISA resource name=w648, write buffer=":MEAS:CURR:DC 2", error in (no error)=w647) -> (VISA resource name out=w645:refnum<visa-resource-name>, error out=w644:errorcluster)  [unwired: 1 out]
                  }
                  frame 3 {
                    n220 = VISA Write(VISA resource name=w653, write buffer=":MEAS:CURR:DC 3", error in (no error)=w652) -> (VISA resource name out=w650:refnum<visa-resource-name>, error out=w649:errorcluster)  [unwired: 1 out]
                  }
                  frame 4 {
                    n221 = VISA Write(VISA resource name=w658, write buffer=":MEAS:CURR:DC 4", error in (no error)=w657) -> (VISA resource name out=w655:refnum<visa-resource-name>, error out=w654:errorcluster)  [unwired: 1 out]
                  }
                  frame 5 {
                    n222 = VISA Write(VISA resource name=w663, write buffer=":MEAS:CURR:DC 5", error in (no error)=w662) -> (VISA resource name out=w660:refnum<visa-resource-name>, error out=w659:errorcluster)  [unwired: 1 out]
                  }
                }
              }
            }
            n223 = local write "Range MAX"(5) -> ()
          }
          frame 2 {
            n224 = stacked-sequence {
              tunnel: w668 -> [_ w678]
              tunnel: w667 -> [_ w677]
              tunnel: [_ w676] -> w666
              tunnel: [_ w675] -> w665
              frame #0 {
                n225 = local read "Range MAX"() -> (w670:dbl)
                n226 = local read "Range No"() -> (w671:dbl)
                n227 = Less?(x=w671, y=w670) -> (x < y?=w672:bool)
                n228 = case shown="True" w672 {
                  frame False {
                  }
                  frame True {
                    n229 = local read "Range No"() -> (w674:dbl)
                    n230 = Increment(x=w674) -> (x+1=w673:dbl)
                    n231 = local write "Range No"(w673) -> ()
                  }
                }
              }
              frame #1 {
                n232 = local read "Range No"() -> (w679:dbl)
                n233 = case shown="4" w679 {
                  tunnel: w678 -> [w684 w689 w694 w699 w704]
                  tunnel: w677 -> [w683 w688 w693 w698 w703]
                  tunnel: [w681 w686 w691 w696 w701] -> w676
                  tunnel: [w680 w685 w690 w695 w700] -> w675
                  frame 0 {
                    n234 = VISA Write(VISA resource name=w684, write buffer=":MEAS:VOLT:AC 0", error in (no error)=w683) -> (VISA resource name out=w681:refnum<visa-resource-name>, error out=w680:errorcluster)  [unwired: 1 out]
                  }
                  frame 1 {
                    n235 = VISA Write(VISA resource name=w689, write buffer=":MEAS:VOLT:AC 1", error in (no error)=w688) -> (VISA resource name out=w686:refnum<visa-resource-name>, error out=w685:errorcluster)  [unwired: 1 out]
                  }
                  frame 2, Default {
                    n236 = VISA Write(VISA resource name=w694, write buffer=":MEAS:VOLT:AC 2", error in (no error)=w693) -> (VISA resource name out=w691:refnum<visa-resource-name>, error out=w690:errorcluster)  [unwired: 1 out]
                  }
                  frame 3 {
                    n237 = VISA Write(VISA resource name=w699, write buffer=":MEAS:VOLT:AC 3", error in (no error)=w698) -> (VISA resource name out=w696:refnum<visa-resource-name>, error out=w695:errorcluster)  [unwired: 1 out]
                  }
                  frame 4 {
                    n238 = VISA Write(VISA resource name=w704, write buffer=":MEAS:VOLT:AC 4", error in (no error)=w703) -> (VISA resource name out=w701:refnum<visa-resource-name>, error out=w700:errorcluster)  [unwired: 1 out]
                  }
                }
              }
            }
            n239 = local write "Range MAX"(4) -> ()
          }
          frame 3 {
            n240 = stacked-sequence {
              tunnel: w709 -> [_ w719]
              tunnel: w708 -> [_ w718]
              tunnel: [_ w717] -> w707
              tunnel: [_ w716] -> w706
              frame #0 {
                n241 = local read "Range MAX"() -> (w711:dbl)
                n242 = local read "Range No"() -> (w712:dbl)
                n243 = Less?(x=w712, y=w711) -> (x < y?=w713:bool)
                n244 = case shown="True" w713 {
                  frame False {
                  }
                  frame True {
                    n245 = local read "Range No"() -> (w715:dbl)
                    n246 = Increment(x=w715) -> (x+1=w714:dbl)
                    n247 = local write "Range No"(w714) -> ()
                  }
                }
              }
              frame #1 {
                n248 = local read "Range No"() -> (w720:dbl)
                n249 = case shown="0" w720 {
                  tunnel: w719 -> [w725 w730 w735 w740]
                  tunnel: w718 -> [w724 w729 w734 w739]
                  tunnel: [w722 w727 w732 w737] -> w717
                  tunnel: [w721 w726 w731 w736] -> w716
                  frame 0 {
                    n250 = VISA Write(VISA resource name=w725, write buffer=":MEAS:CURR:AC 0", error in (no error)=w724) -> (VISA resource name out=w722:refnum<visa-resource-name>, error out=w721:errorcluster)  [unwired: 1 out]
                  }
                  frame 1 {
                    n251 = VISA Write(VISA resource name=w730, write buffer=":MEAS:CURR:AC 1", error in (no error)=w729) -> (VISA resource name out=w727:refnum<visa-resource-name>, error out=w726:errorcluster)  [unwired: 1 out]
                  }
                  frame 2, Default {
                    n252 = VISA Write(VISA resource name=w735, write buffer=":MEAS:CURR:AC 2", error in (no error)=w734) -> (VISA resource name out=w732:refnum<visa-resource-name>, error out=w731:errorcluster)  [unwired: 1 out]
                  }
                  frame 3 {
                    n253 = VISA Write(VISA resource name=w740, write buffer=":MEAS:CURR:AC 3", error in (no error)=w739) -> (VISA resource name out=w737:refnum<visa-resource-name>, error out=w736:errorcluster)  [unwired: 1 out]
                  }
                }
              }
            }
            n254 = local write "Range MAX"(3) -> ()
          }
          frame 4 {
            n255 = stacked-sequence {
              tunnel: w745 -> [_ w755]
              tunnel: w744 -> [_ w754]
              tunnel: [_ w753] -> w743
              tunnel: [_ w752] -> w742
              frame #0 {
                n256 = local read "Range MAX"() -> (w747:dbl)
                n257 = local read "Range No"() -> (w748:dbl)
                n258 = Less?(x=w748, y=w747) -> (x < y?=w749:bool)
                n259 = case shown="True" w749 {
                  frame False {
                  }
                  frame True {
                    n260 = local read "Range No"() -> (w751:dbl)
                    n261 = Increment(x=w751) -> (x+1=w750:dbl)
                    n262 = local write "Range No"(w750) -> ()
                  }
                }
              }
              frame #1 {
                n263 = local read "Range No"() -> (w756:dbl)
                n264 = case shown="1" w756 {
                  tunnel: w755 -> [w761 w766 w771 w776 w781 w786 w791]
                  tunnel: w754 -> [w760 w765 w770 w775 w780 w785 w790]
                  tunnel: [w758 w763 w768 w773 w778 w783 w788] -> w752
                  tunnel: [w757 w762 w767 w772 w777 w782 w787] -> w753
                  frame 0 {
                    n265 = VISA Write(VISA resource name=w761, write buffer=":MEAS:RES 0", error in (no error)=w760) -> (VISA resource name out=w758:refnum<visa-resource-name>, error out=w757:errorcluster)  [unwired: 1 out]
                  }
                  frame 1 {
                    n266 = VISA Write(VISA resource name=w766, write buffer=":MEAS:RES 1", error in (no error)=w765) -> (VISA resource name out=w763:refnum<visa-resource-name>, error out=w762:errorcluster)  [unwired: 1 out]
                  }
                  frame 2, Default {
                    n267 = VISA Write(VISA resource name=w771, write buffer=":MEAS:RES 2", error in (no error)=w770) -> (VISA resource name out=w768:refnum<visa-resource-name>, error out=w767:errorcluster)  [unwired: 1 out]
                  }
                  frame 3 {
                    n268 = VISA Write(VISA resource name=w776, write buffer=":MEAS:RES 3", error in (no error)=w775) -> (VISA resource name out=w773:refnum<visa-resource-name>, error out=w772:errorcluster)  [unwired: 1 out]
                  }
                  frame 4 {
                    n269 = VISA Write(VISA resource name=w781, write buffer=":MEAS:RES 4", error in (no error)=w780) -> (VISA resource name out=w778:refnum<visa-resource-name>, error out=w777:errorcluster)  [unwired: 1 out]
                  }
                  frame 5 {
                    n270 = VISA Write(VISA resource name=w786, write buffer=":MEAS:RES 5", error in (no error)=w785) -> (VISA resource name out=w783:refnum<visa-resource-name>, error out=w782:errorcluster)  [unwired: 1 out]
                  }
                  frame 6 {
                    n271 = VISA Write(VISA resource name=w791, write buffer=":MEAS:RES 6", error in (no error)=w790) -> (VISA resource name out=w788:refnum<visa-resource-name>, error out=w787:errorcluster)  [unwired: 1 out]
                  }
                }
              }
            }
            n272 = local write "Range MAX"(6) -> ()
          }
          frame 5 {
            n273 = stacked-sequence {
              tunnel: w796 -> [_ w806]
              tunnel: w795 -> [_ w805]
              tunnel: [_ w804] -> w794
              tunnel: [_ w803] -> w793
              frame #0 {
                n274 = local read "Range MAX"() -> (w798:dbl)
                n275 = local read "Range No"() -> (w799:dbl)
                n276 = Less?(x=w799, y=w798) -> (x < y?=w800:bool)
                n277 = case shown="True" w800 {
                  frame False {
                  }
                  frame True {
                    n278 = local read "Range No"() -> (w802:dbl)
                    n279 = Increment(x=w802) -> (x+1=w801:dbl)
                    n280 = local write "Range No"(w801) -> ()
                  }
                }
              }
              frame #1 {
                n281 = local read "Range No"() -> (w807:dbl)
                n282 = case shown="6" w807 {
                  tunnel: w806 -> [w812 w817 w822 w827 w832 w837 w842]
                  tunnel: w805 -> [w811 w816 w821 w826 w831 w836 w841]
                  tunnel: [w809 w814 w819 w824 w829 w834 w839] -> w804
                  tunnel: [w808 w813 w818 w823 w828 w833 w838] -> w803
                  frame 0 {
                    n283 = VISA Write(VISA resource name=w812, write buffer=":MEAS:FRES 0", error in (no error)=w811) -> (VISA resource name out=w809:refnum<visa-resource-name>, error out=w808:errorcluster)  [unwired: 1 out]
                  }
                  frame 1 {
                    n284 = VISA Write(VISA resource name=w817, write buffer=":MEAS:FRES 1", error in (no error)=w816) -> (VISA resource name out=w814:refnum<visa-resource-name>, error out=w813:errorcluster)  [unwired: 1 out]
                  }
                  frame 2, Default {
                    n285 = VISA Write(VISA resource name=w822, write buffer=":MEAS:FRES 2", error in (no error)=w821) -> (VISA resource name out=w819:refnum<visa-resource-name>, error out=w818:errorcluster)  [unwired: 1 out]
                  }
                  frame 3 {
                    n286 = VISA Write(VISA resource name=w827, write buffer=":MEAS:FRES 3", error in (no error)=w826) -> (VISA resource name out=w824:refnum<visa-resource-name>, error out=w823:errorcluster)  [unwired: 1 out]
                  }
                  frame 4 {
                    n287 = VISA Write(VISA resource name=w832, write buffer=":MEAS:FRES 4", error in (no error)=w831) -> (VISA resource name out=w829:refnum<visa-resource-name>, error out=w828:errorcluster)  [unwired: 1 out]
                  }
                  frame 5 {
                    n288 = VISA Write(VISA resource name=w837, write buffer=":MEAS:FRES 5", error in (no error)=w836) -> (VISA resource name out=w834:refnum<visa-resource-name>, error out=w833:errorcluster)  [unwired: 1 out]
                  }
                  frame 6 {
                    n289 = VISA Write(VISA resource name=w842, write buffer=":MEAS:FRES 6", error in (no error)=w841) -> (VISA resource name out=w839:refnum<visa-resource-name>, error out=w838:errorcluster)  [unwired: 1 out]
                  }
                }
              }
            }
            n290 = local write "Range MAX"(6) -> ()
          }
          frame 6 {
            n291 = stacked-sequence {
              tunnel: w847 -> [_ w857]
              tunnel: w846 -> [_ w856]
              tunnel: [_ w855] -> w845
              tunnel: [_ w854] -> w844
              frame #0 {
                n292 = local read "Range MAX"() -> (w849:dbl)
                n293 = local read "Range No"() -> (w850:dbl)
                n294 = Less?(x=w850, y=w849) -> (x < y?=w851:bool)
                n295 = case shown="True" w851 {
                  frame False {
                  }
                  frame True {
                    n296 = local read "Range No"() -> (w853:dbl)
                    n297 = Increment(x=w853) -> (x+1=w852:dbl)
                    n298 = local write "Range No"(w852) -> ()
                  }
                }
              }
              frame #1 {
                n299 = local read "Range No"() -> (w858:dbl)
                n300 = case shown="1" w858 {
                  tunnel: w856 -> [w863 w868 w873 w878 w883]
                  tunnel: w857 -> [w862 w867 w872 w877 w882]
                  tunnel: [w860 w865 w870 w875 w880] -> w855
                  tunnel: [w859 w864 w869 w874 w879] -> w854
                  frame 0 {
                    n301 = VISA Write(VISA resource name=w863, write buffer=":MEAS:FREQ 0", error in (no error)=w862) -> (VISA resource name out=w860:refnum<visa-resource-name>, error out=w859:errorcluster)  [unwired: 1 out]
                  }
                  frame 1 {
                    n302 = VISA Write(VISA resource name=w868, write buffer=":MEAS:FREQ 1", error in (no error)=w867) -> (VISA resource name out=w865:refnum<visa-resource-name>, error out=w864:errorcluster)  [unwired: 1 out]
                  }
                  frame 2, Default {
                    n303 = VISA Write(VISA resource name=w873, write buffer=":MEAS:FREQ 2", error in (no error)=w872) -> (VISA resource name out=w870:refnum<visa-resource-name>, error out=w869:errorcluster)  [unwired: 1 out]
                  }
                  frame 3 {
                    n304 = VISA Write(VISA resource name=w878, write buffer=":MEAS:FREQ 3", error in (no error)=w877) -> (VISA resource name out=w875:refnum<visa-resource-name>, error out=w874:errorcluster)  [unwired: 1 out]
                  }
                  frame 4 {
                    n305 = VISA Write(VISA resource name=w883, write buffer=":MEAS:FREQ 4", error in (no error)=w882) -> (VISA resource name out=w880:refnum<visa-resource-name>, error out=w879:errorcluster)  [unwired: 1 out]
                  }
                }
              }
            }
            n306 = local write "Range MAX"(4) -> ()
          }
          frame 7 {
            n307 = stacked-sequence {
              tunnel: w888 -> [_ w898]
              tunnel: w887 -> [_ w897]
              tunnel: [_ w896] -> w886
              tunnel: [_ w895] -> w885
              frame #0 {
                n308 = local read "Range MAX"() -> (w890:dbl)
                n309 = local read "Range No"() -> (w891:dbl)
                n310 = Less?(x=w891, y=w890) -> (x < y?=w892:bool)
                n311 = case shown="True" w892 {
                  frame False {
                  }
                  frame True {
                    n312 = local read "Range No"() -> (w894:dbl)
                    n313 = Increment(x=w894) -> (x+1=w893:dbl)
                    n314 = local write "Range No"(w893) -> ()
                  }
                }
              }
              frame #1 {
                n315 = local read "Range No"() -> (w899:dbl)
                n316 = case shown="0" w899 {
                  tunnel: w897 -> [w904 w909 w914 w919 w924]
                  tunnel: w898 -> [w903 w908 w913 w918 w923]
                  tunnel: [w901 w906 w911 w916 w921] -> w896
                  tunnel: [w900 w905 w910 w915 w920] -> w895
                  frame 0 {
                    n317 = VISA Write(VISA resource name=w904, write buffer=":MEAS:PER 0", error in (no error)=w903) -> (VISA resource name out=w901:refnum<visa-resource-name>, error out=w900:errorcluster)  [unwired: 1 out]
                  }
                  frame 1 {
                    n318 = VISA Write(VISA resource name=w909, write buffer=":MEAS:PER 1", error in (no error)=w908) -> (VISA resource name out=w906:refnum<visa-resource-name>, error out=w905:errorcluster)  [unwired: 1 out]
                  }
                  frame 2, Default {
                    n319 = VISA Write(VISA resource name=w914, write buffer=":MEAS:PER 2", error in (no error)=w913) -> (VISA resource name out=w911:refnum<visa-resource-name>, error out=w910:errorcluster)  [unwired: 1 out]
                  }
                  frame 3 {
                    n320 = VISA Write(VISA resource name=w919, write buffer=":MEAS:PER 3", error in (no error)=w918) -> (VISA resource name out=w916:refnum<visa-resource-name>, error out=w915:errorcluster)  [unwired: 1 out]
                  }
                  frame 4 {
                    n321 = VISA Write(VISA resource name=w924, write buffer=":MEAS:PER 4", error in (no error)=w923) -> (VISA resource name out=w921:refnum<visa-resource-name>, error out=w920:errorcluster)  [unwired: 1 out]
                  }
                }
              }
            }
            n322 = local write "Range MAX"(4) -> ()
          }
          frame 8 {
            n323 = stacked-sequence {
              tunnel: w929 -> [_ w939]
              tunnel: w928 -> [_ w938]
              tunnel: [_ w937] -> w927
              tunnel: [_ w936] -> w926
              frame #0 {
                n324 = local read "Range MAX"() -> (w931:dbl)
                n325 = local read "Range No"() -> (w932:dbl)
                n326 = Less?(x=w932, y=w931) -> (x < y?=w933:bool)
                n327 = case shown="True" w933 {
                  frame False {
                  }
                  frame True {
                    n328 = local read "Range No"() -> (w935:dbl)
                    n329 = Increment(x=w935) -> (x+1=w934:dbl)
                    n330 = local write "Range No"(w934) -> ()
                  }
                }
              }
              frame #1 {
                n331 = local read "Range No"() -> (w940:dbl)
                n332 = case shown="0" w940 {
                  tunnel: w938 -> [w945 w950 w955 w960 w965]
                  tunnel: w939 -> [w944 w949 w954 w959 w964]
                  tunnel: [w942 w947 w952 w957 w962] -> w937
                  tunnel: [w941 w946 w951 w956 w961] -> w936
                  frame 0 {
                    n333 = VISA Write(VISA resource name=w945, write buffer=":MEAS:VOLT:DC 0", error in (no error)=w944) -> (VISA resource name out=w942:refnum<visa-resource-name>, error out=w941:errorcluster)  [unwired: 1 out]
                  }
                  frame 1 {
                    n334 = VISA Write(VISA resource name=w950, write buffer=":MEAS:VOLT:DC 1", error in (no error)=w949) -> (VISA resource name out=w947:refnum<visa-resource-name>, error out=w946:errorcluster)  [unwired: 1 out]
                  }
                  frame 2, Default {
                    n335 = VISA Write(VISA resource name=w955, write buffer=":MEAS:VOLT:DC 2", error in (no error)=w954) -> (VISA resource name out=w952:refnum<visa-resource-name>, error out=w951:errorcluster)  [unwired: 1 out]
                  }
                  frame 3 {
                    n336 = VISA Write(VISA resource name=w960, write buffer=":MEAS:VOLT:DC 3", error in (no error)=w959) -> (VISA resource name out=w957:refnum<visa-resource-name>, error out=w956:errorcluster)  [unwired: 1 out]
                  }
                  frame 4 {
                    n337 = VISA Write(VISA resource name=w965, write buffer=":MEAS:VOLT:DC 4", error in (no error)=w964) -> (VISA resource name out=w962:refnum<visa-resource-name>, error out=w961:errorcluster)  [unwired: 1 out]
                  }
                }
              }
            }
            n338 = local write "Range MAX"(4) -> ()
          }
          frame 9 {
            n339 = stacked-sequence {
              tunnel: [_ w980] -> w970
              tunnel: [_ w979] -> w969
              tunnel: w968 -> [_ w978]
              tunnel: w967 -> [_ w977]
              frame #0 {
                n340 = local read "Range MAX"() -> (w972:dbl)
                n341 = local read "Range No"() -> (w973:dbl)
                n342 = Less?(x=w973, y=w972) -> (x < y?=w974:bool)
                n343 = case shown="True" w974 {
                  frame False {
                  }
                  frame True {
                    n344 = local read "Range No"() -> (w976:dbl)
                    n345 = Increment(x=w976) -> (x+1=w975:dbl)
                    n346 = local write "Range No"(w975) -> ()
                  }
                }
              }
              frame #1 {
                n347 = local read "Range No"() -> (w981:dbl)
                n348 = case shown="5" w981 {
                  tunnel: w977 -> [w986 w991 w996 w1001 w1006 w1011]
                  tunnel: w978 -> [w985 w990 w995 w1000 w1005 w1010]
                  tunnel: [w983 w988 w993 w998 w1003 w1008] -> w980
                  tunnel: [w982 w987 w992 w997 w1002 w1007] -> w979
                  frame 0 {
                    n349 = VISA Write(VISA resource name=w986, write buffer=":MEAS:CAP 0", error in (no error)=w985) -> (VISA resource name out=w983:refnum<visa-resource-name>, error out=w982:errorcluster)  [unwired: 1 out]
                  }
                  frame 1 {
                    n350 = VISA Write(VISA resource name=w991, write buffer=":MEAS:CAP 1", error in (no error)=w990) -> (VISA resource name out=w988:refnum<visa-resource-name>, error out=w987:errorcluster)  [unwired: 1 out]
                  }
                  frame 2, Default {
                    n351 = VISA Write(VISA resource name=w996, write buffer=":MEAS:CAP 2", error in (no error)=w995) -> (VISA resource name out=w993:refnum<visa-resource-name>, error out=w992:errorcluster)  [unwired: 1 out]
                  }
                  frame 3 {
                    n352 = VISA Write(VISA resource name=w1001, write buffer=":MEAS:CAP 3", error in (no error)=w1000) -> (VISA resource name out=w998:refnum<visa-resource-name>, error out=w997:errorcluster)  [unwired: 1 out]
                  }
                  frame 4 {
                    n353 = VISA Write(VISA resource name=w1006, write buffer=":MEAS:CAP 4", error in (no error)=w1005) -> (VISA resource name out=w1003:refnum<visa-resource-name>, error out=w1002:errorcluster)  [unwired: 1 out]
                  }
                  frame 5 {
                    n354 = VISA Write(VISA resource name=w1011, write buffer=":MEAS:CAP 5", error in (no error)=w1010) -> (VISA resource name out=w1008:refnum<visa-resource-name>, error out=w1007:errorcluster)  [unwired: 1 out]
                  }
                }
              }
            }
            n355 = local write "Range MAX"(5) -> ()
          }
          frame 10 {
            n356 = stacked-sequence {
              tunnel: [_ w1026] -> w1016
              tunnel: [_ w1025] -> w1015
              tunnel: w1014 -> [_ w1024]
              tunnel: w1013 -> [_ w1023]
              frame #0 {
                n357 = local read "Range MAX"() -> (w1018:dbl)
                n358 = local read "Range No"() -> (w1019:dbl)
                n359 = Less?(x=w1019, y=w1018) -> (x < y?=w1020:bool)
                n360 = case shown="True" w1020 {
                  frame False {
                  }
                  frame True {
                    n361 = local read "Range No"() -> (w1022:dbl)
                    n362 = Increment(x=w1022) -> (x+1=w1021:dbl)
                    n363 = local write "Range No"(w1021) -> ()
                  }
                }
              }
              frame #1 {
                n364 = local read "Range No"() -> (w1027:dbl)
                n365 = case shown="2, Default" w1027 {
                  tunnel: w1024 -> [w1032 w1037 w1042 w1047 w1052]
                  tunnel: w1023 -> [w1031 w1036 w1041 w1046 w1051]
                  tunnel: [w1029 w1034 w1039 w1044 w1049] -> w1026
                  tunnel: [w1028 w1033 w1038 w1043 w1048] -> w1025
                  frame 0 {
                    n366 = VISA Write(VISA resource name=w1032, write buffer=":MEAS:VOLT:DC 0", error in (no error)=w1031) -> (VISA resource name out=w1029:refnum<visa-resource-name>, error out=w1028:errorcluster)  [unwired: 1 out]
                  }
                  frame 1 {
                    n367 = VISA Write(VISA resource name=w1037, write buffer=":MEAS:VOLT:DC 1", error in (no error)=w1036) -> (VISA resource name out=w1034:refnum<visa-resource-name>, error out=w1033:errorcluster)  [unwired: 1 out]
                  }
                  frame 2, Default {
                    n368 = VISA Write(VISA resource name=w1042, write buffer=":MEAS:VOLT:DC 2", error in (no error)=w1041) -> (VISA resource name out=w1039:refnum<visa-resource-name>, error out=w1038:errorcluster)  [unwired: 1 out]
                  }
                  frame 3 {
                    n369 = VISA Write(VISA resource name=w1047, write buffer=":MEAS:VOLT:DC 3", error in (no error)=w1046) -> (VISA resource name out=w1044:refnum<visa-resource-name>, error out=w1043:errorcluster)  [unwired: 1 out]
                  }
                  frame 4 {
                    n370 = VISA Write(VISA resource name=w1052, write buffer=":MEAS:VOLT:DC 4", error in (no error)=w1051) -> (VISA resource name out=w1049:refnum<visa-resource-name>, error out=w1048:errorcluster)  [unwired: 1 out]
                  }
                }
              }
            }
            n371 = local write "Range MAX"(4) -> ()
          }
        }
      }
      event "Measure": Value Change {
        n372 = event-data() -> ()  [unwired: 1 in, 6 out]
        n373 = case shown="2" w1054 {
          selector: w1054 -> [w1060 w1078 w1096 w1114 w1132 w1150 w1168 w1186 w1204 w1222 w1240]
          tunnel: w1056 -> [w1061 w1080 w1098 w1116 w1134 w1151 w1170 w1191 w1206 w1227 w1242]
          tunnel: w1059 -> [w1062 w1079 w1097 w1115 w1133 w1152 w1169 w1190 w1205 w1226 w1241]
          tunnel: [w1064 w1081 w1099 w1118 w1136 w1154 w1172 w1188 w1208 w1224 w1244] -> w1058
          tunnel: [w1065 w1083 w1101 w1119 w1137 w1155 w1173 w1189 w1209 w1225 w1245] -> w1057
          tunnel: [w1063 w1082 w1100 w1117 w1135 w1153 w1171 w1187 w1207 w1223 w1243] -> w1055
          tunnel: [w1060 w1078 w1096 w1114 w1132 w1150 w1168 w1186 w1204 w1222 w1240] -> w1053
          frame 0, Default {
            n374 = stacked-sequence {
              seq-local: [w1067 _] -> [_ w1075]
              tunnel: w1061 -> [w1068 w1076]
              tunnel: [_ w1074] -> w1065
              tunnel: [_ w1073] -> w1064
              tunnel: [_ w1072] -> w1063
              tunnel: w1062 -> [w1066 w1071]
              frame #0 {
                n375 = Wait (ms)(milliseconds to wait=u32 100) -> ()  [unwired: 1 out]
                n376 = VISA Write(VISA resource name=w1068, write buffer=":MEAS:VOLT:DC? ", error in (no error)=w1066) -> (return count=w1067:u32)  [unwired: 2 out]
              }
              frame #1 {
                n377 = Wait (ms)(milliseconds to wait=u32 100) -> ()  [unwired: 1 out]
                n378 = VISA Read(VISA resource name=w1076, byte count=w1075, error in (no error)=w1071) -> (VISA resource name out=w1074:refnum<visa-resource-name>, read buffer=w1072:string, error out=w1073:errorcluster)  [unwired: 1 out]
              }
            }
          }
          frame 1 {
            n379 = stacked-sequence {
              seq-local: [w1084 _] -> [_ w1092]
              tunnel: w1080 -> [w1086 w1094]
              tunnel: w1079 -> [w1085 w1093]
              tunnel: [_ w1091] -> w1083
              tunnel: [_ w1090] -> w1081
              tunnel: [_ w1089] -> w1082
              frame #0 {
                n380 = Wait (ms)(milliseconds to wait=u32 100) -> ()  [unwired: 1 out]
                n381 = VISA Write(VISA resource name=w1086, write buffer=":MEASure:CURR:DC? ", error in (no error)=w1085) -> (return count=w1084:u32)  [unwired: 2 out]
              }
              frame #1 {
                n382 = Wait (ms)(milliseconds to wait=u32 100) -> ()  [unwired: 1 out]
                n383 = VISA Read(VISA resource name=w1094, byte count=w1092, error in (no error)=w1093) -> (VISA resource name out=w1091:refnum<visa-resource-name>, read buffer=w1089:string, error out=w1090:errorcluster)  [unwired: 1 out]
              }
            }
          }
          frame 2 {
            n384 = stacked-sequence {
              seq-local: [w1103 _] -> [_ w1111]
              tunnel: w1097 -> [w1104 w1112]
              tunnel: [_ w1110] -> w1101
              tunnel: [_ w1109] -> w1100
              tunnel: w1098 -> [w1102 w1108]
              tunnel: [_ w1107] -> w1099
              frame #0 {
                n385 = Wait (ms)(milliseconds to wait=u32 100) -> ()  [unwired: 1 out]
                n386 = VISA Write(VISA resource name=w1102, write buffer=":MEAS:VOLT:AC? ", error in (no error)=w1104) -> (return count=w1103:u32)  [unwired: 2 out]
              }
              frame #1 {
                n387 = Wait (ms)(milliseconds to wait=u32 100) -> ()  [unwired: 1 out]
                n388 = VISA Read(VISA resource name=w1108, byte count=w1111, error in (no error)=w1112) -> (VISA resource name out=w1110:refnum<visa-resource-name>, read buffer=w1109:string, error out=w1107:errorcluster)  [unwired: 1 out]
              }
            }
          }
          frame 3 {
            n389 = stacked-sequence {
              seq-local: [w1122 _] -> [_ w1130]
              tunnel: [_ w1129] -> w1119
              tunnel: [_ w1128] -> w1118
              tunnel: [_ w1127] -> w1117
              tunnel: w1116 -> [w1121 w1125]
              tunnel: w1115 -> [w1120 w1126]
              frame #0 {
                n390 = Wait (ms)(milliseconds to wait=u32 100) -> ()  [unwired: 1 out]
                n391 = VISA Write(VISA resource name=w1121, write buffer=":MEASure:CURR:AC? ", error in (no error)=w1120) -> (return count=w1122:u32)  [unwired: 2 out]
              }
              frame #1 {
                n392 = Wait (ms)(milliseconds to wait=u32 100) -> ()  [unwired: 1 out]
                n393 = VISA Read(VISA resource name=w1125, byte count=w1130, error in (no error)=w1126) -> (VISA resource name out=w1129:refnum<visa-resource-name>, read buffer=w1127:string, error out=w1128:errorcluster)  [unwired: 1 out]
              }
            }
          }
          frame 4 {
            n394 = stacked-sequence {
              seq-local: [w1138 _] -> [_ w1146]
              tunnel: w1134 -> [w1140 w1148]
              tunnel: w1133 -> [w1139 w1147]
              tunnel: [_ w1145] -> w1137
              tunnel: [_ w1144] -> w1136
              tunnel: [_ w1143] -> w1135
              frame #0 {
                n395 = Wait (ms)(milliseconds to wait=u32 100) -> ()  [unwired: 1 out]
                n396 = VISA Write(VISA resource name=w1140, write buffer=":MEASure:RES? ", error in (no error)=w1139) -> (return count=w1138:u32)  [unwired: 2 out]
              }
              frame #1 {
                n397 = Wait (ms)(milliseconds to wait=u32 100) -> ()  [unwired: 1 out]
                n398 = VISA Read(VISA resource name=w1148, byte count=w1146, error in (no error)=w1147) -> (VISA resource name out=w1145:refnum<visa-resource-name>, read buffer=w1143:string, error out=w1144:errorcluster)  [unwired: 1 out]
              }
            }
          }
          frame 5 {
            n399 = stacked-sequence {
              seq-local: [w1156 _] -> [_ w1164]
              tunnel: w1151 -> [w1158 w1166]
              tunnel: w1152 -> [w1157 w1165]
              tunnel: [_ w1163] -> w1155
              tunnel: [_ w1162] -> w1154
              tunnel: [_ w1161] -> w1153
              frame #0 {
                n400 = Wait (ms)(milliseconds to wait=u32 100) -> ()  [unwired: 1 out]
                n401 = VISA Write(VISA resource name=w1158, write buffer=":MEASure:FRES? ", error in (no error)=w1157) -> (return count=w1156:u32)  [unwired: 2 out]
              }
              frame #1 {
                n402 = Wait (ms)(milliseconds to wait=u32 100) -> ()  [unwired: 1 out]
                n403 = VISA Read(VISA resource name=w1166, byte count=w1164, error in (no error)=w1165) -> (VISA resource name out=w1163:refnum<visa-resource-name>, read buffer=w1161:string, error out=w1162:errorcluster)  [unwired: 1 out]
              }
            }
          }
          frame 6 {
            n404 = stacked-sequence {
              seq-local: [w1174 _] -> [_ w1182]
              tunnel: w1170 -> [w1176 w1184]
              tunnel: w1169 -> [w1175 w1183]
              tunnel: [_ w1181] -> w1173
              tunnel: [_ w1180] -> w1172
              tunnel: [_ w1179] -> w1171
              frame #0 {
                n405 = Wait (ms)(milliseconds to wait=u32 100) -> ()  [unwired: 1 out]
                n406 = VISA Write(VISA resource name=w1176, write buffer=":MEASure:FREQ? ", error in (no error)=w1175) -> (return count=w1174:u32)  [unwired: 2 out]
              }
              frame #1 {
                n407 = Wait (ms)(milliseconds to wait=u32 100) -> ()  [unwired: 1 out]
                n408 = VISA Read(VISA resource name=w1184, byte count=w1182, error in (no error)=w1183) -> (VISA resource name out=w1181:refnum<visa-resource-name>, read buffer=w1179:string, error out=w1180:errorcluster)  [unwired: 1 out]
              }
            }
          }
          frame 7 {
            n409 = stacked-sequence {
              seq-local: [w1192 _] -> [_ w1200]
              tunnel: w1191 -> [w1194 w1202]
              tunnel: w1190 -> [w1193 w1201]
              tunnel: [_ w1199] -> w1189
              tunnel: [_ w1198] -> w1188
              tunnel: [_ w1197] -> w1187
              frame #0 {
                n410 = Wait (ms)(milliseconds to wait=u32 100) -> ()  [unwired: 1 out]
                n411 = VISA Write(VISA resource name=w1194, write buffer=":MEASure:PER? ", error in (no error)=w1193) -> (return count=w1192:u32)  [unwired: 2 out]
              }
              frame #1 {
                n412 = Wait (ms)(milliseconds to wait=u32 100) -> ()  [unwired: 1 out]
                n413 = VISA Read(VISA resource name=w1202, byte count=w1200, error in (no error)=w1201) -> (VISA resource name out=w1199:refnum<visa-resource-name>, read buffer=w1197:string, error out=w1198:errorcluster)  [unwired: 1 out]
              }
            }
          }
          frame 8 {
            n414 = stacked-sequence {
              seq-local: [w1210 _] -> [_ w1218]
              tunnel: w1206 -> [w1212 w1220]
              tunnel: w1205 -> [w1211 w1219]
              tunnel: [_ w1217] -> w1209
              tunnel: [_ w1216] -> w1208
              tunnel: [_ w1215] -> w1207
              frame #0 {
                n415 = Wait (ms)(milliseconds to wait=u32 100) -> ()  [unwired: 1 out]
                n416 = VISA Write(VISA resource name=w1212, write buffer=":MEASure:DIOD? ", error in (no error)=w1211) -> (return count=w1210:u32)  [unwired: 2 out]
              }
              frame #1 {
                n417 = Wait (ms)(milliseconds to wait=u32 100) -> ()  [unwired: 1 out]
                n418 = VISA Read(VISA resource name=w1220, byte count=w1218, error in (no error)=w1219) -> (VISA resource name out=w1217:refnum<visa-resource-name>, read buffer=w1215:string, error out=w1216:errorcluster)  [unwired: 1 out]
              }
            }
          }
          frame 9 {
            n419 = stacked-sequence {
              seq-local: [w1228 _] -> [_ w1236]
              tunnel: w1227 -> [w1230 w1238]
              tunnel: w1226 -> [w1229 w1237]
              tunnel: [_ w1235] -> w1225
              tunnel: [_ w1234] -> w1224
              tunnel: [_ w1233] -> w1223
              frame #0 {
                n420 = Wait (ms)(milliseconds to wait=u32 100) -> ()  [unwired: 1 out]
                n421 = VISA Write(VISA resource name=w1230, write buffer=":MEASure:CAP? ", error in (no error)=w1229) -> (return count=w1228:u32)  [unwired: 2 out]
              }
              frame #1 {
                n422 = Wait (ms)(milliseconds to wait=u32 100) -> ()  [unwired: 1 out]
                n423 = VISA Read(VISA resource name=w1238, byte count=w1236, error in (no error)=w1237) -> (VISA resource name out=w1235:refnum<visa-resource-name>, read buffer=w1233:string, error out=w1234:errorcluster)  [unwired: 1 out]
              }
            }
          }
          frame 10 {
            n424 = stacked-sequence {
              seq-local: [w1246 _] -> [_ w1254]
              tunnel: w1242 -> [w1248 w1256]
              tunnel: w1241 -> [w1247 w1255]
              tunnel: [_ w1253] -> w1245
              tunnel: [_ w1252] -> w1244
              tunnel: [_ w1251] -> w1243
              frame #0 {
                n425 = Wait (ms)(milliseconds to wait=u32 100) -> ()  [unwired: 1 out]
                n426 = VISA Write(VISA resource name=w1248, write buffer=":MEASure:CONT? ", error in (no error)=w1247) -> (return count=w1246:u32)  [unwired: 2 out]
              }
              frame #1 {
                n427 = Wait (ms)(milliseconds to wait=u32 100) -> ()  [unwired: 1 out]
                n428 = VISA Read(VISA resource name=w1256, byte count=w1254, error in (no error)=w1255) -> (VISA resource name out=w1253:refnum<visa-resource-name>, read buffer=w1251:string, error out=w1252:errorcluster)  [unwired: 1 out]
              }
            }
          }
        }
      }
    }
    n429 = Insert Into Array(array=w6, new element=w10) -> (w7:string[])  [unwired: 1 in]
    "Results, V" <- w7
    n430 = VISA Close(VISA resource name=w11, error in (no error)=w12) -> (error out=→"error out":errorcluster)
  }
  "Range No" <- 1.0 ("Range No")
